vi "Check and Expand Array.vi"(1 "?":dbl[][](array[numeric]) format="%.2f") -> (0 "?":dbl[][](array[numeric]) format="%.2f")   [LabVIEW 2020]
panel:
  in  "Case Constant\n(See Context Help)":bool
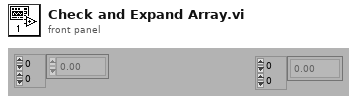
[diagram p1: front panel]
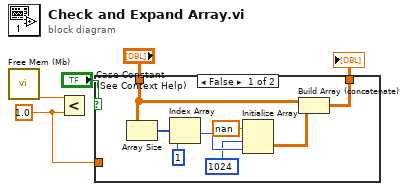
[diagram p0: block diagram]
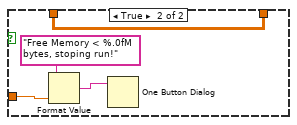
[diagram p2: hidden frame]
diagram:
  w4 = 1.0
  n1 = call "Free Mem (Mb).vi"() -> ("Free Memory (Mb)"=w5:dbl)
  n2 = Less?(x=w5, y=w4) -> ()  [unwired: 1 out]
  n3 = case shown="False" "Case Constant\n(See Context Help)" {
    tunnel: w4 -> [_ w15]
    tunnel: "?" -> [w7 w14]
    tunnel: [w6 w14] -> w2
    frame False {
      n4 = Array Size(array=w7) -> (size(s)=w13:i32[])
      n5 = Index Array(array=w13, index=1) -> (element=w11:i32)
      n6 = Initialize Array(nan, 1024, w11) -> (w8:dbl[][])
      n7 = Build Array (concatenate)(w7, w8) -> (w6:dbl[][])
    }
    frame True {
      n8 = Format Value(format string="Free Memory < %.0fM bytes, stoping run!", value (0)=w15) -> (output string=w17:string)  [unwired: 1 in]
      n9 = One Button Dialog(message=w17) -> ()  [unwired: 1 in, 1 out]
    }
  }
  "?" <- w2
